vi "Set CAN Publishing.vi"(5 "Box ID":u8=1, 7 "DIO":bool, 8 "error in (no error)":errorcluster, 9 "AI":bool, 10 "AO":bool, 11 "BS120x in":refnum<class "BS120x.lvclass">) -> (0 "error out":errorcluster, 3 "BS120x out":refnum<class "BS120x.lvclass">)   [LabVIEW 2021, in "BS120x Driver.lvlib" / "BS120x.lvclass"]
uses:
  BS120x.lvclass
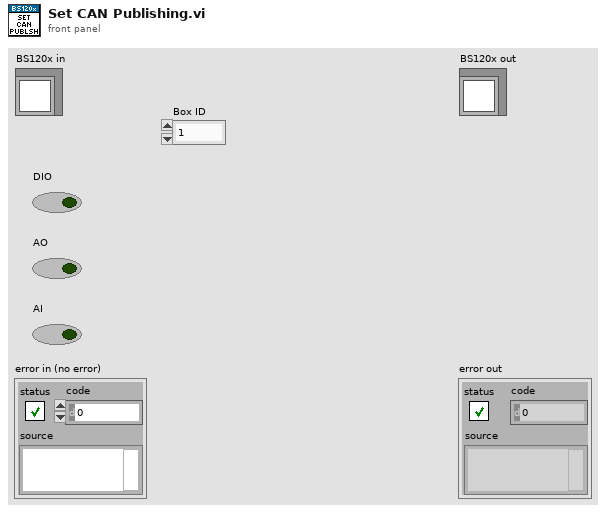
[diagram p1: front panel]
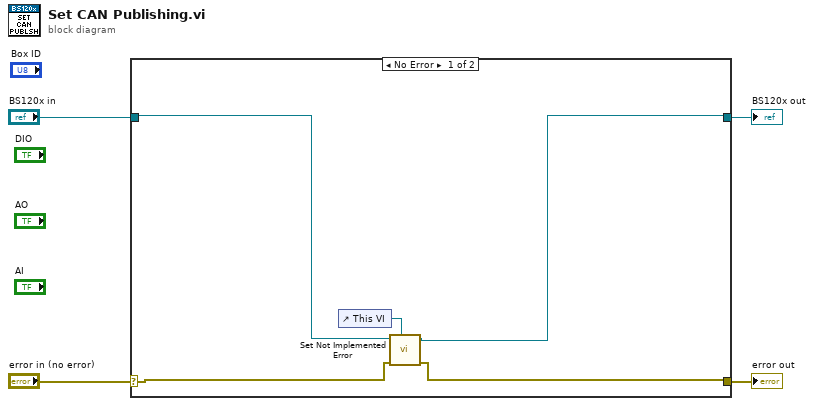
[diagram p0: block diagram]
diagram:
  n1 = case shown="No Error" "error in (no error)" {
    selector: "error in (no error)" -> [w7 w11]
    tunnel: [w5 w11] -> w3
    tunnel: [w6 w10] -> w1
    tunnel: "BS120x in" -> [w8 w10]
    frame No Error {
      n2 = control-ref of="This VI"() -> (w9:refnum<vi>)
      n3 = call "Set Not Implemented Error.vi"("VI Reference"=w9, "error in (no error)"=w7, "BS120x in"=w8) -> ("error out"=w5:errorcluster, "BS120x out"=w6:refnum<class "BS120x.lvclass">)  [unwired: 7 in]
    }
    frame Error {
    }
  }
  "error out" <- w3
  "BS120x out" <- w1
